vi "Generator.GetPrivateEvents.vi"(8 "error in (no error)":errorcluster, 11 "Generator":refnum<class "Generator.lvclass">) -> (0 "error out":errorcluster, 2 "Generator Private Events":T1, 3 "Generator out":refnum<class "Generator.lvclass">)   [LabVIEW 2019, in "Generator.lvclass"]
doc: "---------------------------------------------------------------\nJKI State Machine Objects™\nhttp://jki.net/state-machine-objects/\nCopyright (C) 2005-2015, JKI <info@jki.net>\nALL RIGHTS RESERVEDJKI State Machine Objects (SMO) 1.0.0.4\nJKI - JKI\nCopyright (c) 2015, JKI"
uses:
  Generator.lvclass
  typedefs/PrivateEvents--Cluster.ctl
  typedefs/Message--Cluster.ctl
  typedefs/Sampling--Cluster.ctl
  typedefs/AO.Channel--Cluster--Array.ctl
  typedefs/AO.Channel--Cluster.ctl
  typedefs/AO.Channel.Function--Enum.ctl
  typedefs/REF.Channel--Cluster--Array.ctl
  typedefs/REF.Channel--Cluster.ctl
  typedefs/Sweep.Configuration--Cluster.ctl
  typedefs/Sweep.Channel--Cluster--Array.ctl
  typedefs/Sweep.Channel--Cluster.ctl
  typedefs/Sweep.Pattern--Enum.ctl
  typedefs/Generator.Command--enum.ctl
  typedefs/WaveformQueues--Cluster.ctl
  Generator.lvclass/Generator.ctl
panel:
  # "For instructions on how to use the JKI State Machine Objects, examples and video tutorials, visit:\nhttp://jki.net/state-machine-objects/\n\nJKI State Machine Objects™\nhttp://jki.net/state-machine-objects/\nCopyright (C) 2005-2015, JKI <info@jki.net>\nALL RIGHTS RESERVED"
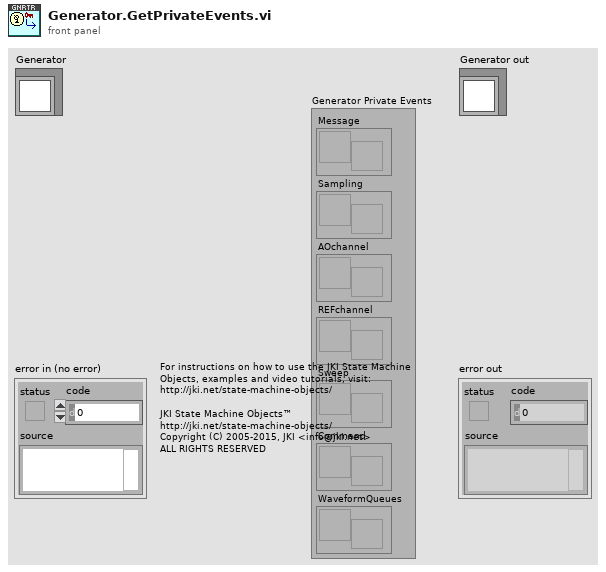
[diagram p1: front panel]
types:
  T1 = typedef "Generator.lvclass/PrivateEvents--Cluster.ctl" = cluster{"Message":refnum<user-event>, "Sampling":refnum<user-event>, "AOchannel":refnum<user-event>, "REFchannel":refnum<user-event>, "Sweep":refnum<user-event>, "Command":refnum<user-event>, "WaveformQueues":refnum<user-event>}
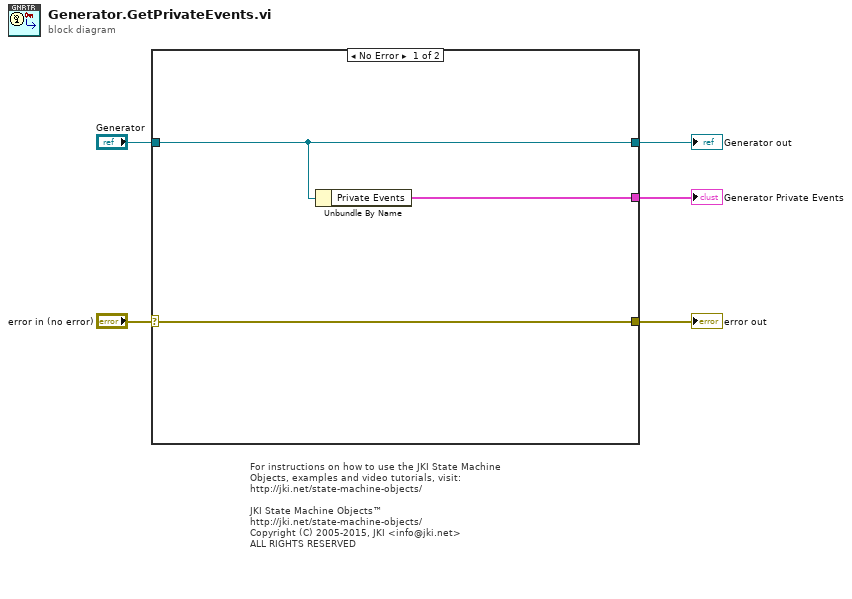
[diagram p0: block diagram]
diagram:
  # "For instructions on how to use the JKI State Machine Objects, examples and video tutorials, visit:\nhttp://jki.net/state-machine-objects/\n\nJKI State Machine Objects™\nhttp://jki.net/state-machine-objects/\nCopyright (C) 2005-2015, JKI <info@jki.net>\nALL RIGHTS RESERVED"
  n1 = case shown="No Error" "error in (no error)" {
    selector: "error in (no error)" -> [w7 w9]
    tunnel: "Generator" -> [w6 w10]
    tunnel: [w7 w9] -> w4
    tunnel: [w6 w10] -> w3
    tunnel: [w8 _] -> w1
    frame No Error {
      n2 = Unbundle By Name(w6) -> ("Private Events"=w8:T1)
    }
    frame Error {
    }
  }
  "error out" <- w4
  "Generator out" <- w3
  "Generator Private Events" <- w1
